vi "saveImage.vi"() -> ()   [LabVIEW 2016]
uses:
  <vilib>/picture/picture.llb/imagedata.ctl
  <vilib>/vision/NI_Vision_Development_Module.lvlib
panel:
  in  "path to BMP file":path
  in  "Chart":refnum<k7>
  in  "Document":refnum<k7>
  in  "Application":refnum<k7>
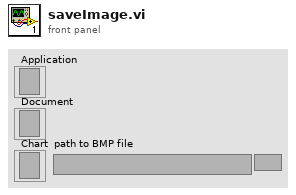
[diagram p1: front panel]
types:
  T1 = typedef "imagedata.ctl" = cluster{"image type":i32, "image depth":i32, "image":u8[], "mask":u8[], "colors":u32[], "Rectangle":cluster{"left":i16, "top":i16, "right":i16, "bottom":i16}}
  T2 = typedef "LVRectTypeDef.ctl" = cluster{"Left":i16, "Top":i16, "Right":i16, "Bottom":i16}
  T3 = typedef "IMAQ Image.ctl" = refnum<image>
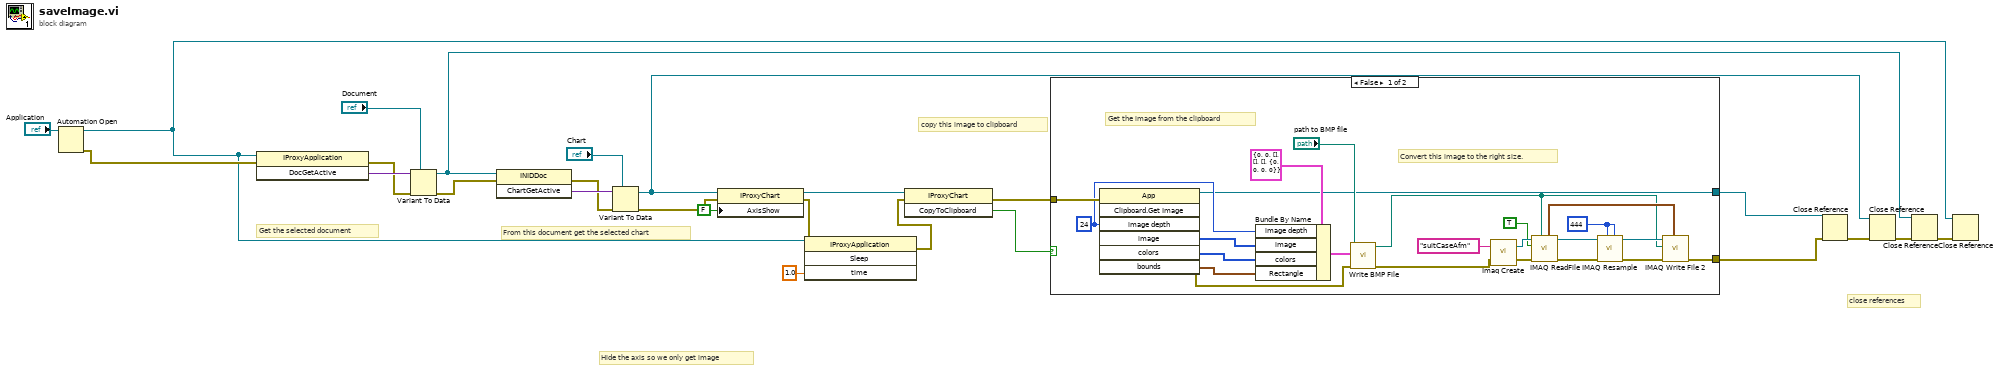
[diagram p0: block diagram]
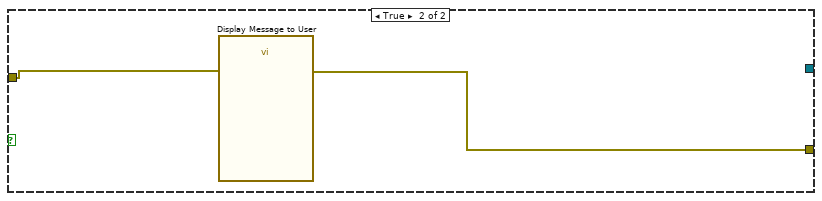
[diagram p2: hidden frame]
diagram:
  # "close references"
  # "copy this image to clipboard"
  # "Hide the axis so we only get image"
  # "From this document get the selected chart"
  # "Get the selected document"
  n1 = Automation Open(Automation Refnum="Application") -> (Automation Refnum=w4:refnum<k7>, error out=w17:errorcluster)  [unwired: 3 in]
  n2 = invoke class="IProxyApplication" method="DocGetActive"(reference=w4, error in=w17) -> (error out=w18:errorcluster, "DocGetActive"=w23:variant)  [unwired: 1 in, 1 out]
  n3 = Variant To Data(error in=w18, type="Document", Variant=w23) -> (data=w5:refnum<k7>, error out=w20:errorcluster)
  n4 = invoke class="INIDDoc" method="ChartGetActive"(reference=w5, error in=w20) -> (error out=w19:errorcluster, "ChartGetActive"=w22:variant)  [unwired: 1 in, 1 out]
  n5 = Variant To Data(error in=w19, type="Chart", Variant=w22) -> (data=w6:refnum<k7>, error out=w13:errorcluster)
  n6 = property class="IProxyChart"(reference=w6, error in=w13, "AxisShow"=FALSE) -> (reference out=w14:refnum<k7>, error out=w2:errorcluster)
  n7 = invoke class="IProxyApplication" method="Sleep"(reference=w4, error in=w2, "time"=1.0) -> (error out=w1:errorcluster)  [unwired: 1 in, 3 out]
  n8 = invoke class="IProxyChart" method="CopyToClipboard"(reference=w14, error in=w1) -> (error out=w15:errorcluster, "CopyToClipboard"=w16:bool)  [unwired: 1 in, 1 out]
  n9 = case shown="False" w16 {
    tunnel: w15 -> [w48 w50]
    tunnel: [w27 w49] -> w11
    tunnel: [w26 _] -> w7
    frame False {
      w35 = 444 ("Y Resolution")
      w43 = 24 ("Image Depth")
      # "Convert this image to the right size."
      # "Get the image from the clipboard"
      n10 = invoke class="App" method="Clipboard.Get Image"(error in=w48, "image depth"=w43) -> (reference out=w26:refnum<vi>, error out=w44:errorcluster, "image"=w45:u8[], "colors"=w42:u32[], "bounds"=w41:T2)  [unwired: 5 in, 2 out]
      n11 = Bundle By Name(cluster=T1 {"image type"=0, "image depth"=0, "image"=[], "mask"=[], "colors"=[], "Rectangle"={"left"=0, "top"=0, "right"=0, "bottom"=0}} ("image data"), "image depth"=w43, "image"=w45, "colors"=w42, "Rectangle"=w41) -> (w46:T1)
      n12 = call <vilib>:"Write BMP File.vi"("error in (no error)"=w44, "image data"=w46, "path to BMP file"="path to BMP file") -> ("error out"=w28:errorcluster, "path"=w29:path)  [unwired: 7 in]
      n13 = call "Imaq Create"("Image Name"="suitCaseAfm", "error in (no error)"=w28) -> ("New Image"=w34:T3, "error out"=w33:errorcluster)  [unwired: 3 in]
      n14 = call "IMAQ ReadFile"("File Path"=w29, "error in (no error)"=w33, "Load Color Palette? (No)"=TRUE, "Image"=w34) -> ("error out"=w38:errorcluster, "Image Out"=w39:T3, "Color Palette out"=w30:cluster{"Red":u8, "Green":u8, "Blue":u8}[])  [unwired: 3 in, 2 out]
      n15 = call "IMAQ Resample"("X Resolution"=w35, "Y Resolution"=w35, "error in (no error)"=w38, "Image Src"=w39) -> ("error out"=w36:errorcluster, "Image Dst Out"=w37:T3)  [unwired: 6 in]
      n16 = call-poly "IMAQ Write File 2"("Color Palette"=w30, "error in (no error)"=w36, "File Path"=w29, "Image"=w37) -> ("error out"=w27:errorcluster)  [unwired: 6 in, 1 out]
    }
    frame True {
      n17 = call "Display Message to User"("error in (no error)"=w50) -> ("error out"=w49:errorcluster)  [unwired: 9 in, 1 out]
    }
  }
  n18 = Close Reference(reference=w7, error in (no error)=w11) -> (error out=w10:errorcluster)
  n19 = Close Reference(reference=w6, error in (no error)=w10) -> (error out=w9:errorcluster)
  n20 = Close Reference(reference=w5, error in (no error)=w9) -> (error out=w8:errorcluster)
  n21 = Close Reference(reference=w4, error in (no error)=w8) -> ()  [unwired: 1 out]
